vi "FdxCmdRxControlCvi.vi"(8 "error in":errorcluster, 9 "GlobalStatisticReset":u32(ring) items=["FDX_RX_GS_RES_NO_CNT", "FDX_RX_GS_RES_ALL_CNT", "FDX_RX_GS_RES_ERR_CNT "], 10 "StartMode":u32(ring)=1 items=["FDX_STOP", "FDX_START"], 11 "InstrumentHandle_port in":u32) -> (0 "error out":errorcluster, 3 "InstrumentHandle_port out":u32)   [LabVIEW 2020, in "AIM664LV.lvlib"]
doc: "This function is used to control the receive operation of the board."
uses:
  AIM664LV.lvlib
  AFDX_LibraryAdmin/FdxGlobalDllPath.vi
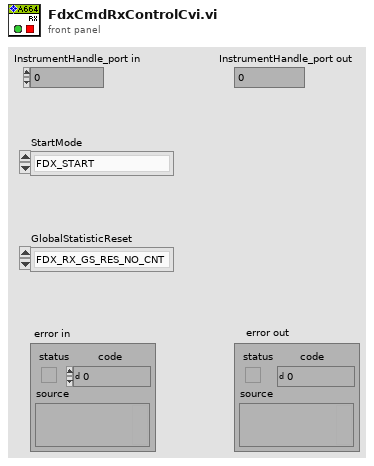
[diagram p1: front panel]
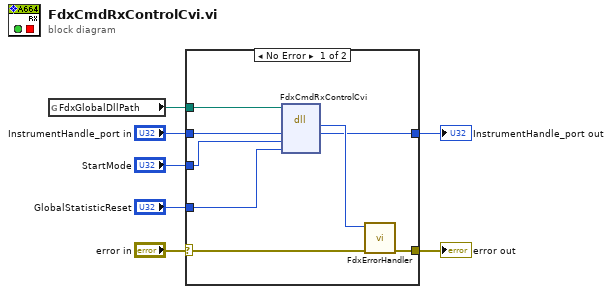
[diagram p0: block diagram]
diagram:
  n1 = global read "FdxGlobalDllPath.vi" "FdxGlobalDllPath"() -> (w5:path)
  n2 = case shown="No Error" "error in" {
    selector: "error in" -> [w14 w17]
    tunnel: [w15 w17] -> w7
    tunnel: w5 -> [w12 _]
    tunnel: "InstrumentHandle_port in" -> [w11 w16]
    tunnel: [w10 w16] -> w3
    tunnel: "StartMode" -> [w9 _]
    tunnel: "GlobalStatisticReset" -> [w8 _]
    frame No Error {
      n3 = dll-call lib="aim_fdx.19.dll" fn="FdxCmdRxControlCvi"(path in=w12, "InstrumentHandle"=w11, "StartMode"=w9, "GlobalStatisticReset"=w8) -> ("status"=w13:i32, "InstrumentHandle"=w10:u32)  [unwired: 4 in, 2 out]
      n4 = call "FdxErrorHandler.vi"("error in"=w14, "AIM Error"=w13) -> ("error out"=w15:errorcluster)  [unwired: 9 in]
    }
    frame Error {
    }
  }
  "error out" <- w7
  "InstrumentHandle_port out" <- w3
